vi "SHA256Time.vi"() -> ()   [LabVIEW 2024]
uses:
  <vilib>/OPCUA/controls/NodeId.ctl
  <vilib>/OPCUA/client/Multiple Read Double.vi
  <vilib>/OPCUA/NI OPC UA Client.lvlib
  <vilib>/Analysis/NI_AALBase.lvlib
panel:
  out "StdDev":dbl format="%0.2f"
  out "Current\nValue":dbl format="%#_15g"
  out "Tolerance, %":dbl
  out "Max-Min":dbl
  out "min value":dbl format="%#_14f"
  out "max value":dbl format="%#_14f"
  out "Average":dbl format="%_14f"
  out "SHA256\nExecution Time":dbl(graph)
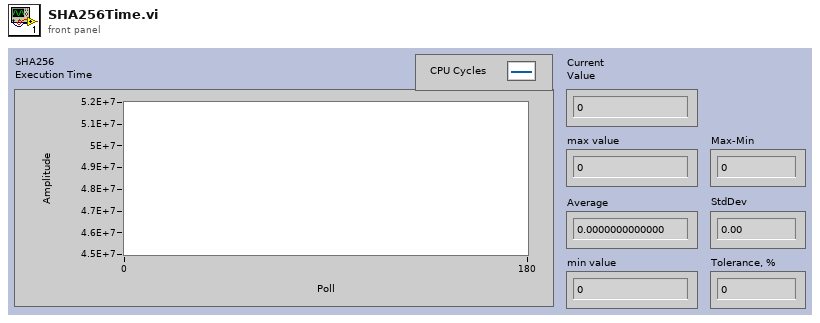
[diagram p1: front panel]
types:
  T1 = typedef "NodeId.ctl" = string
  T2 = typedef "OPC UA Client Refnum.ctl" = refnum<k21>
  T3 = typedef "OPC UA StatusCode.ctl" = u32
  T4 = cluster{"node ID":T1, "value ":dbl, "timestamp":timestamp, "status":T3}[]
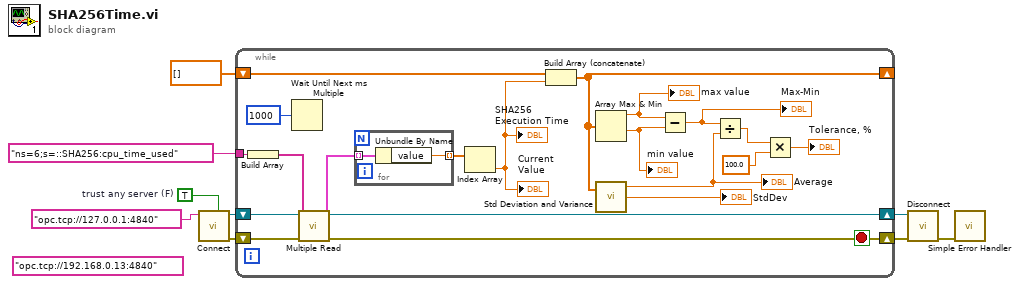
[diagram p0: block diagram]
diagram:
  (unwired) "opc.tcp://192.168.0.13:4840" ("server endpoint URL")
  w7 = TRUE  # trust any server (F)
  n1 = call <vilib>:"Connect.vi"("trust any server (F)"=w7, "server endpoint URL"="opc.tcp://127.0.0.1:4840") -> ("error out"=w3:errorcluster, "OPC UA client refnum out"=w6:T2)  [unwired: 7 in, 1 out]
  n2 = while {
    shift-right: [w28] -> w5
    shift-left: w6 -> [w26]
    shift-right: [w23] -> _
    shift-left: dbl[] [] -> [w24]
    shift-right: [w13] -> w2
    shift-left: w3 -> [w14]
    tunnel: T1 "ns=6;s=::SHA256:cpu_time_used" ("node RU") -> [w11]
    stop <- w13 stop-if-true
    n3 = Build Array(w11) -> (w10:T1[])
    n4 = Wait Until Next ms Multiple(millisecond multiple=u32 1000) -> ()  [unwired: 1 out]
    n5 = call-poly <vilib>:"Multiple Read.vi"("error in (no error)"=w14, "node IDs"=w10, "OPC UA client refnum in"=w26) -> ("error out"=w13:errorcluster, "results"=w29:T4, "OPC UA client refnum out"=w28:T2)  [unwired: 5 in, 1 out]
    n6 = for {
      tunnel: w29 -> [w31] mode=indexing
      tunnel: [w30] -> w25 mode=indexing
      n7 = Unbundle By Name(w31) -> ("value"=w30:dbl)
    }
    n8 = Index Array(array=w25) -> (element=w15:dbl)  [unwired: 1 in]
    "SHA256\nExecution Time" <- w15
    "Current\nValue" <- w15
    n9 = Build Array (concatenate)(w24, w15) -> (w23:dbl[])
    n10 = Array Max & Min(array=w23) -> (max value=w22:dbl, min value=w21:dbl)  [unwired: 2 out]
    "max value" <- w22
    "min value" <- w21
    n11 = call <vilib>:"Std Deviation and Variance.vi"("X"=w23) -> ("mean"=w19:dbl, "standard deviation"=→"StdDev":dbl)  [unwired: 1 in, 1 out]
    "Average" <- w19
    n12 = Subtract(x=w22, y=w21) -> (x-y=w20:dbl)
    "Max-Min" <- w20
    n13 = Divide(x=w20, y=w19) -> (x/y=w18:dbl)
    n14 = Multiply(x=w18, y=100.0) -> (x*y=→"Tolerance, %":dbl)
  }
  n15 = call <vilib>:"Disconnect.vi"("error in (no error)"=w2, "OPC UA client refnum in"=w5) -> ("error out"=w9:errorcluster)  [unwired: 9 in]
  n16 = call <vilib>:"Simple Error Handler.vi"("error in (no error)"=w9) -> ()  [unwired: 4 in, 5 out]
